vi "Binomial Inverse CDF.vi"(9 "p":dbl=0.02, 10 "n":i32=1, 11 "cdf(x)":dbl=0.5) -> (0 "error":i32, 3 "x":i32)   [LabVIEW 2020, in "NI_Gmath.lvlib"]
doc: "Computes the discrete inverse cumulative distribution function (CDF), or the value <B>x</B> such that the probability that the random variate X, where X describes the selected distribution type, takes on a value less than or equal to it is <B>cdf(x)</B>. You must manually select the polymorphic instance to use."
uses:
  <vilib>/gmath/NI_Gmath.lvlib
panel:
  # "Binomial Inverse CDF"
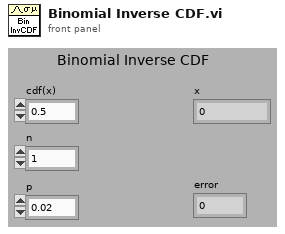
[diagram p1: front panel]
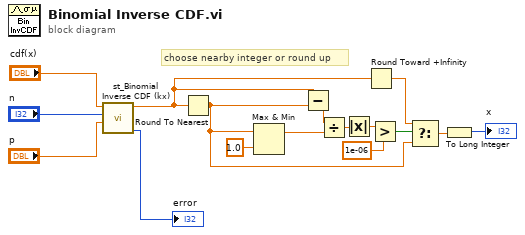
[diagram p0: block diagram]
diagram:
  # "choose nearby integer or round up"
  n1 = call <vilib>:"st_Binomial Inverse CDF (kx).vi"("p"="p", "n"="n", "cdf(x)"="cdf(x)") -> ("error"=→"error":i32, "x"=w4:dbl)  [unwired: 7 in]
  n2 = Round To Nearest(number=w4) -> (nearest integer value=w3:dbl)
  n3 = Max & Min(x=w3, y=1.0) -> (max(x,y)=w2:dbl)  [unwired: 1 out]
  n4 = Subtract(x=w4, y=w3) -> (x-y=w15:dbl)
  n5 = Divide(x=w15, y=w2) -> (x/y=w13:dbl)
  n6 = Absolute Value(x=w13) -> (abs(x)=w14:dbl)
  n7 = Round Toward +Infinity(x=w4) -> (ceil(x): smallest int >= x=w10:dbl)
  n8 = Greater?(x=w14, y=1e-06) -> (0:w11:bool)
  n9 = Select(t=w10, s=w11, f=w3) -> (s? t:f=w16:dbl)
  n10 = To Long Integer(number=w16) -> (32bit integer=→"x":i32)
